vi "Handle Command.vi"(8 "error in (no error)":errorcluster, 9 "Data":variant, 10 "Command":string, 11 "instrument.PPMS in":refnum<class "instrument.PPMS3.lvclass">) -> (0 "error out":errorcluster, 1 "Processed Data":variant, 2 "Command":string, 3 "instrument.PPMS out":refnum<class "instrument.PPMS3.lvclass">)   [LabVIEW 2016, in "instrument.PPMS3.lvclass"]
uses:
  instrument.PPMS3.lvclass
  Typedefs/PPMS.Magnet Field--cluster.ctl
  Typedefs/PPMS.Temperature--cluster.ctl
  <userlib>/LevyLab/Levylab Instruments/Instrument Types/Cryostat/Typedefs/Magnet Mode--Enum.ctl
  <userlib>/LevyLab/Levylab Instruments/Instrument Types/Cryostat/Instrument.Cryostat.lvclass
  Typedefs/PPMS.Magnet Status--cluster.ctl
  Typedefs/PPMS.Temperature Status--cluster.ctl
  instrument.PPMS/instrument.PPMS.lvclass
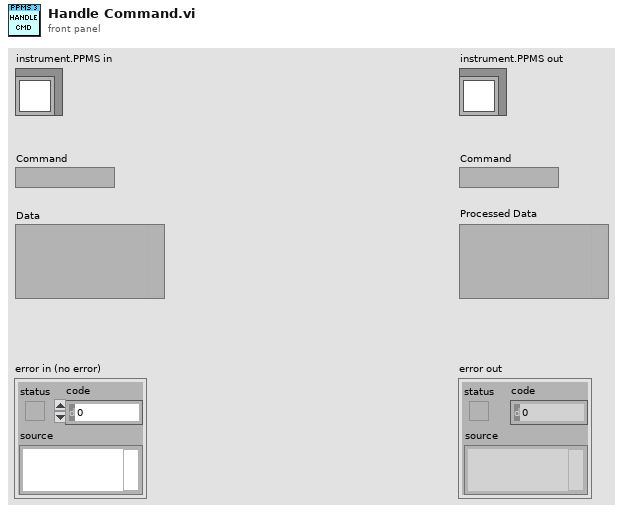
[diagram p1: front panel]
types:
  T1 = typedef "instrument.PPMS3.lvclass/PPMS.Temperature--cluster.ctl" = cluster{"Temperature (K)":dbl, "Rate (K/min)":dbl}
  T2 = typedef "instrument.PPMS3.lvclass/PPMS.Magnet Field--cluster.ctl" = cluster{"Target Field (Oe)":dbl, "Target Rate (Oe/s)":dbl, "Mode":T3}
  T3 = typedef "Instrument.Cryostat.lvclass/Magnet Mode--Enum.ctl" = enum16{"Persistent", "Driven"}
  T4 = typedef "instrument.PPMS3.lvclass/PPMS.Magnet Status--cluster.ctl" = cluster{"Field (Oe)":dbl, "Magnet Status":string}
  T5 = typedef "instrument.PPMS3.lvclass/PPMS.Temperature Status--cluster.ctl" = cluster{"Temperature (K)":dbl, "Temperature Status":string}
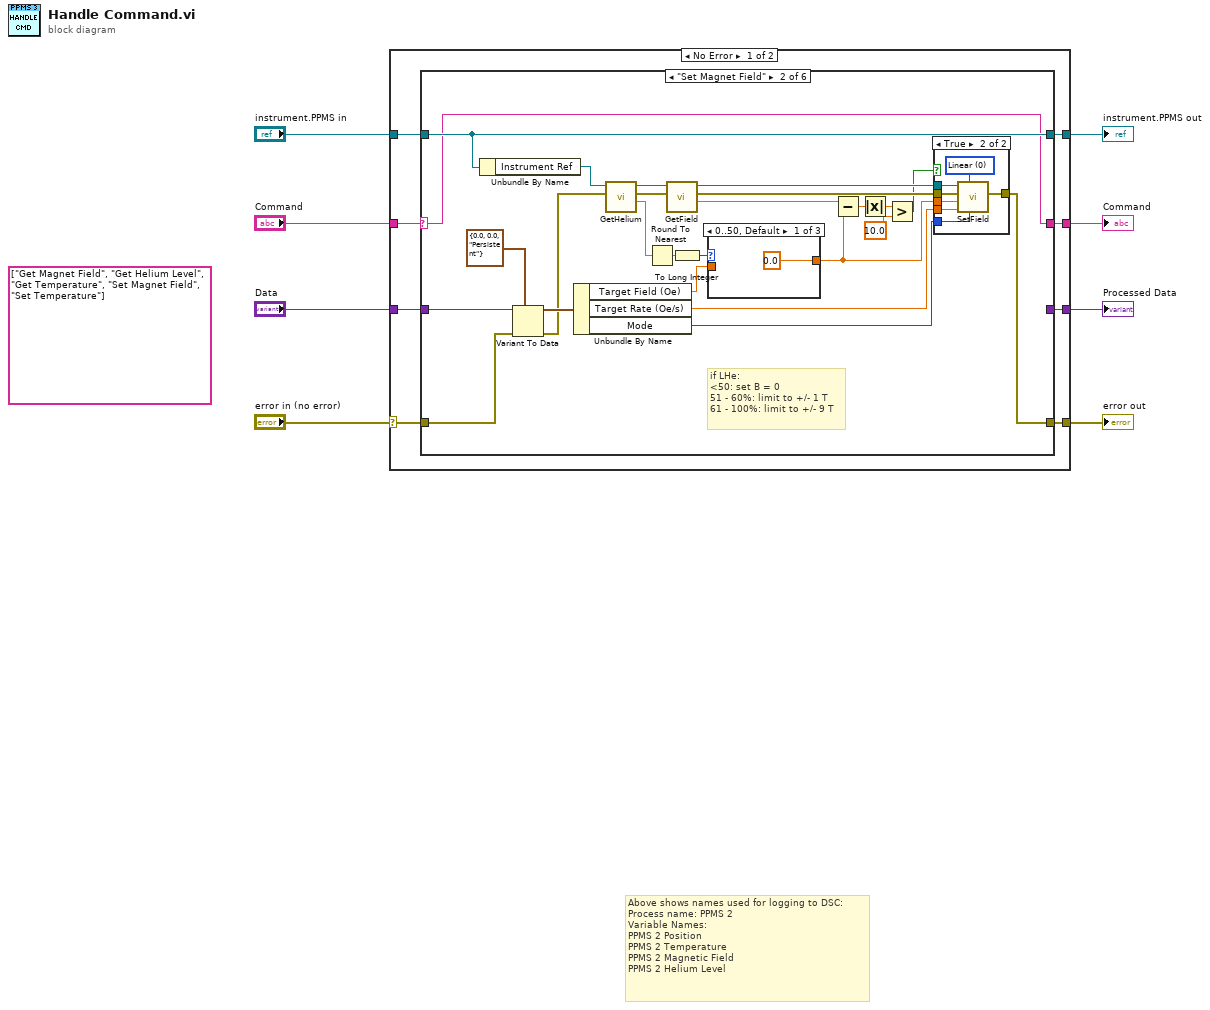
[diagram p0: block diagram]
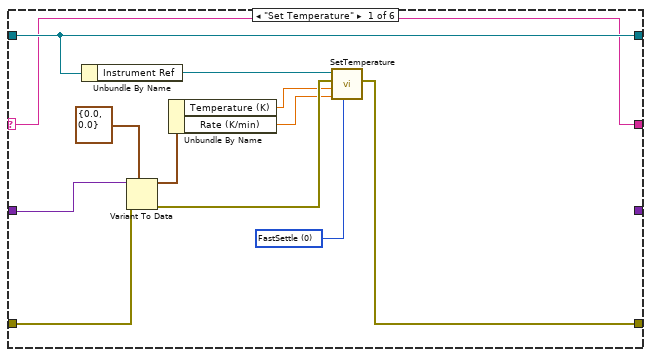
[diagram p2: hidden frame]
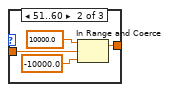
[diagram p3: hidden frame]
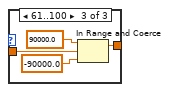
[diagram p4: hidden frame]
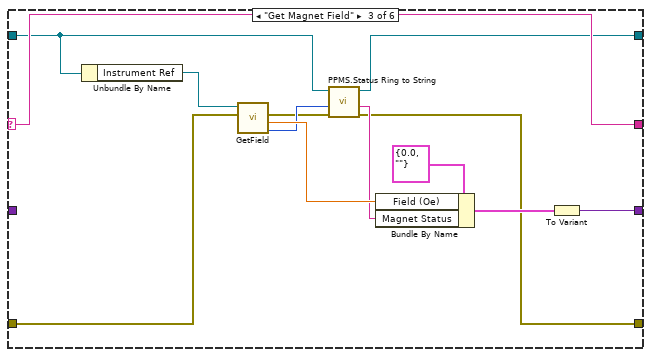
[diagram p6: hidden frame]
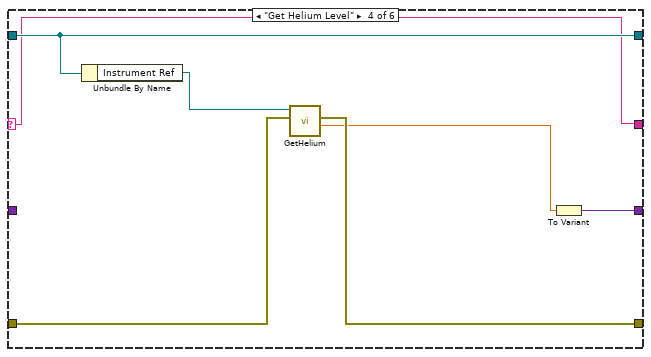
[diagram p7: hidden frame]
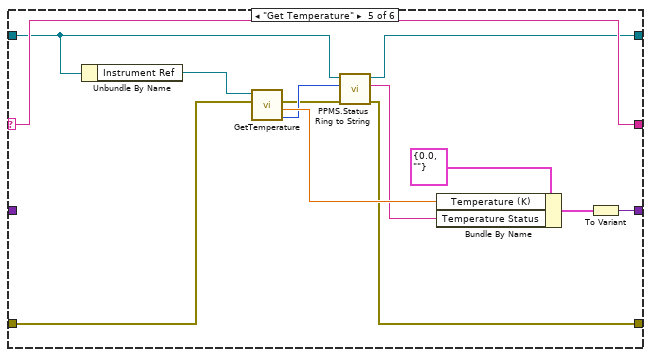
[diagram p8: hidden frame]
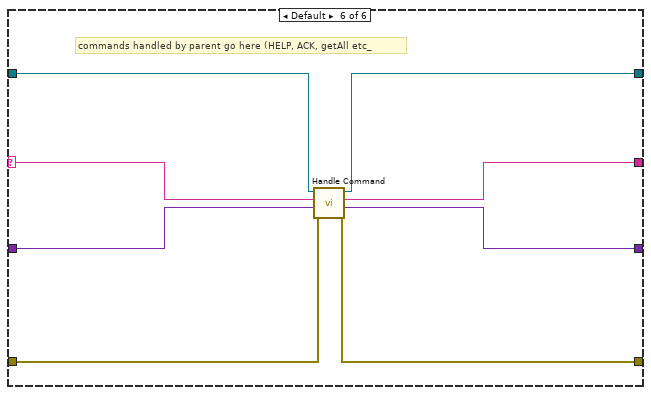
[diagram p9: hidden frame]
diagram:
  (unwired) string[] ["Get Magnet Field", "Get Helium Level", "Get Temperature", "Set Magnet Field", "Set Temperature"] ("Commands")
  # "Above shows names used for logging to DSC:\nProcess name: PPMS 2\nVariable Names:\nPPMS 2 Position\nPPMS 2 Temperature\nPPMS 2 Magnetic Field\nPPMS 2 Helium Level"
  n1 = case shown="No Error" "error in (no error)" {
    selector: "error in (no error)" -> [w11 w112]
    tunnel: [w10 w112] -> w6
    tunnel: [w16 _] -> w4
    tunnel: [w15 _] -> w5
    tunnel: [w14 w113] -> w7
    tunnel: "Data" -> [w13 _]
    tunnel: "Command" -> [w9 _]
    tunnel: "instrument.PPMS in" -> [w12 w113]
    frame No Error {
      n2 = case shown="\"Set Magnet Field\"" w9 {
        selector: w9 -> [w17 w35 w77 w84 w97 w104]
        tunnel: [_ _ w78 w86 w101 w111] -> w16
        tunnel: [w17 w35 w77 w84 w97 w110] -> w15
        tunnel: [w28 w53 w71 w90 w94 w109] -> w14
        tunnel: w13 -> [w23 w51 _ _ _ w108]
        tunnel: w12 -> [w28 w53 w72 w90 w95 w107]
        tunnel: w11 -> [w25 w50 w82 w89 w102 w106]
        tunnel: [w26 w48 w73 w88 w92 w105] -> w10
        frame "Set Temperature" {
          w18 = 0 items=["FastSettle", "NoOvershoot"] ("Approach")
          n3 = Unbundle By Name(w28) -> ("Instrument Ref"=w27:refnum<k24>)
          n4 = Variant To Data(error in=w25, type=T1 {"Temperature (K)"=0.0, "Rate (K/min)"=0.0} ("Temperature"), Variant=w23) -> (data=w22:T1, error out=w21:errorcluster)
          n5 = Unbundle By Name(w22) -> ("Temperature (K)"=w20:dbl, "Rate (K/min)"=w19:dbl)
          n6 = call "SetTemperature.vi"("Approach"=w18, "Rate"=w19, "Temperature"=w20, "error in (no error)"=w21, "Instrument Ref In"=w27) -> ("error out"=w26:errorcluster)  [unwired: 2 in, 2 out]
        }
        frame "Set Magnet Field" {
          # "if LHe:\n<50: set B = 0\n51 - 60%: limit to +/- 1 T\n61 - 100%: limit to +/- 9 T"
          n7 = Unbundle By Name(w53) -> ("Instrument Ref"=w34:refnum<k24>)
          n8 = Variant To Data(error in=w50, type=T2 {"Target Field (Oe)"=0.0, "Target Rate (Oe/s)"=0.0, "Mode"=enum."Persistent"} ("Magnet Field"), Variant=w51) -> (data=w49:T2, error out=w47:errorcluster)
          n9 = Unbundle By Name(w49) -> ("Target Field (Oe)"=w41:dbl, "Target Rate (Oe/s)"=w42:dbl, "Mode"=w36:T3)
          n10 = call "GetHelium.vi"("error in (no error)"=w47, "Instrument Refnum in"=w34) -> ("Helium Level (%)"=w32:dbl, "error out"=w46:errorcluster, "Instrument Ref Out"=w44:refnum<k24>)  [unwired: 3 in]
          n11 = Round To Nearest(number=w32) -> (nearest integer value=w31:dbl)
          n12 = call "GetField.vi"("error in (no error)"=w46, "Instrument Ref In"=w44) -> ("Field"=w38:dbl, "error out"=w45:errorcluster, "Instrument Ref Out"=w43:refnum<k24>)  [unwired: 3 in, 2 out]
          n13 = To Long Integer(number=w31) -> (32bit integer=w30:i32)
          n14 = case shown="0..50, Default" w30 {
            tunnel: w41 -> [_ w56 w60]
            tunnel: [0.0 ("upper limit") w55 w59] -> w33
            frame 0..50, Default {
            }
            frame 51..60 {
              n15 = In Range and Coerce(upper limit=10000.0, x=w56, lower limit=-10000.0) -> (coerced(x)=w55:dbl)  [unwired: 1 out]
            }
            frame 61..100 {
              n16 = In Range and Coerce(upper limit=90000.0, x=w60, lower limit=-90000.0) -> (coerced(x)=w59:dbl)  [unwired: 1 out]
            }
          }
          n17 = Subtract(x=w38, y=w33) -> (x-y=w37:dbl)
          n18 = Absolute Value(x=w37) -> (abs(x)=w40:dbl)
          n19 = Greater?(x=w40, y=10.0) -> (0:w29:bool)
          n20 = case shown="True" w29 {
            tunnel: [w63 w69] -> w48
            tunnel: w45 -> [w63 w68]
            tunnel: w43 -> [_ w67]
            tunnel: w42 -> [_ w66]
            tunnel: w33 -> [_ w65]
            tunnel: w36 -> [_ w64]
            frame False {
            }
            frame True {
              w70 = 0 items=["Linear", "NoOvershoot", "Oscillate"] ("Approach")
              n21 = call "SetField.vi"("Mode"=w64, "Approach"=w70, "Rate"=w66, "Field"=w65, "error in (no error)"=w68, "Instrument Ref In"=w67) -> ("error out"=w69:errorcluster)  [unwired: 1 in, 2 out]
            }
          }
        }
        frame "Get Magnet Field" {
          n22 = Unbundle By Name(w72) -> ("Instrument Ref"=w83:refnum<k24>)
          n23 = call "GetField.vi"("error in (no error)"=w82, "Instrument Ref In"=w83) -> ("Field\nStatus"=w76:i32, "Field"=w81:dbl, "error out"=w74:errorcluster)  [unwired: 3 in, 2 out]
          n24 = call "PPMS.Status Ring to String.vi"("error in (no error)"=w74, "Field Status"=w76, "instrument.PPMS in"=w72) -> ("error out"=w73:errorcluster, "Field Status String"=w75:string, "instrument.PPMS out"=w71:refnum<class "instrument.PPMS3.lvclass">)  [unwired: 5 in, 1 out]
          n25 = Bundle By Name(cluster=T4 {"Field (Oe)"=0.0, "Magnet Status"=""}, "Field (Oe)"=w81, "Magnet Status"=w75) -> (w79:T4)
          n26 = To Variant(anything=w79) -> (Variant=w78:variant)
        }
        frame "Get Helium Level" {
          n27 = Unbundle By Name(w90) -> ("Instrument Ref"=w85:refnum<k24>)
          n28 = call "GetHelium.vi"("error in (no error)"=w89, "Instrument Refnum in"=w85) -> ("Helium Level (%)"=w87:dbl, "error out"=w88:errorcluster)  [unwired: 3 in, 1 out]
          n29 = To Variant(anything=w87) -> (Variant=w86:variant)
        }
        frame "Get Temperature" {
          n30 = Unbundle By Name(w95) -> ("Instrument Ref"=w103:refnum<k24>)
          n31 = call "GetTemperature.vi"("error in (no error)"=w102, "Instrument Ref In"=w103) -> ("Temperature\nStatus"=w96:i32, "Temperature"=w100:dbl, "error out"=w93:errorcluster)  [unwired: 3 in, 2 out]
          n32 = call "PPMS.Status Ring to String.vi"("error in (no error)"=w93, "Temperature Status"=w96, "instrument.PPMS in"=w95) -> ("error out"=w92:errorcluster, "Temperature Status String"=w91:string, "instrument.PPMS out"=w94:refnum<class "instrument.PPMS3.lvclass">)  [unwired: 5 in, 1 out]
          n33 = Bundle By Name(cluster=T5 {"Temperature (K)"=0.0, "Temperature Status"=""}, "Temperature (K)"=w100, "Temperature Status"=w91) -> (w98:T5)
          n34 = To Variant(anything=w98) -> (Variant=w101:variant)
        }
        frame Default {
          # "commands handled by parent go here (HELP, ACK, getAll etc_"
          n35 = call-parent "Handle Command.vi"("error in (no error)"=w106, "Data"=w108, "Command"=w104, "instrument.PPMS in"=w107) -> ("error out"=w105:errorcluster, "Processed Data"=w111:variant, "Command"=w110:string, "instrument.PPMS out"=w109:refnum<class "instrument.PPMS3.lvclass">)  [unwired: 4 in]
        }
      }
    }
    frame Error {
    }
  }
  "error out" <- w6
  "instrument.PPMS out" <- w7
  "Processed Data" <- w4
  "Command" <- w5
